vi "case structure.vi"() -> ()   [LabVIEW 2025]
panel:
  out "output":string
  in  "B":dbl
  in  "A":dbl
  out "Numeric":dbl
  in  "String 3":string
  out "month":string
  in  "month in num":dbl
  out "String":string
  in  "OK Button":bool
  in  "stop":bool
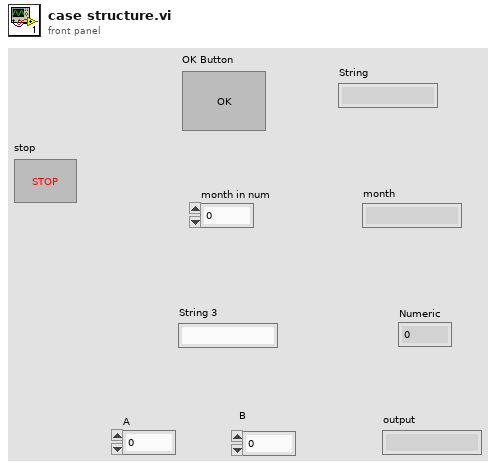
[diagram p1: front panel]
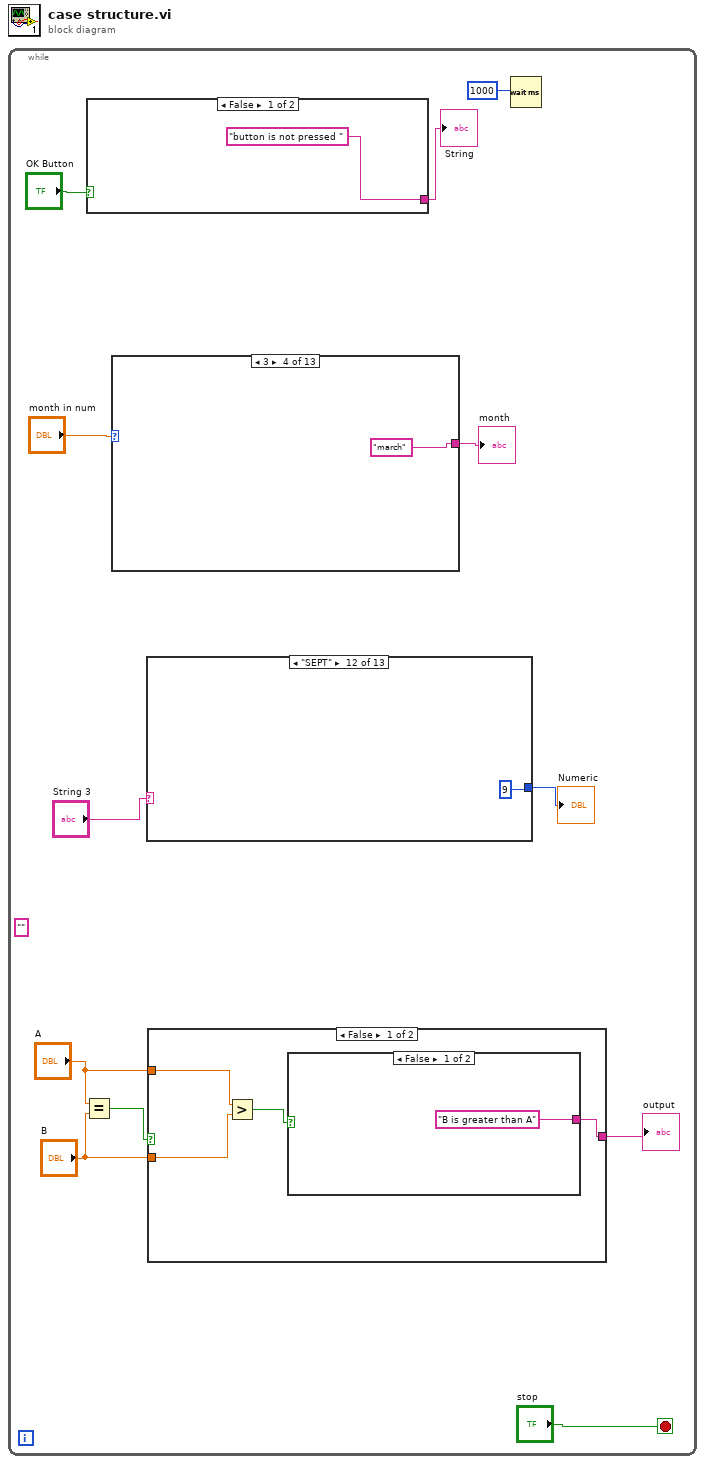
[diagram p0: block diagram]
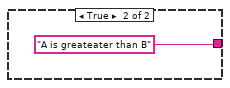
[diagram p2: hidden frame]
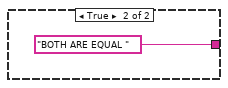
[diagram p3: hidden frame]
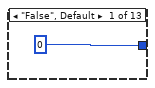
[diagram p4: hidden frame]
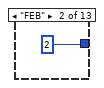
[diagram p5: hidden frame]
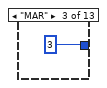
[diagram p6: hidden frame]
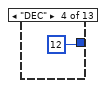
[diagram p7: hidden frame]
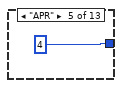
[diagram p8: hidden frame]
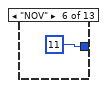
[diagram p9: hidden frame]
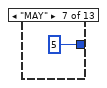
[diagram p10: hidden frame]
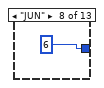
[diagram p11: hidden frame]
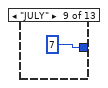
[diagram p12: hidden frame]
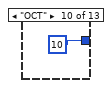
[diagram p13: hidden frame]
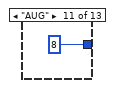
[diagram p14: hidden frame]
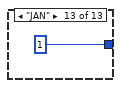
[diagram p15: hidden frame]
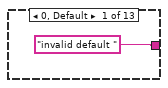
[diagram p16: hidden frame]
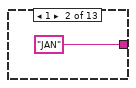
[diagram p17: hidden frame]
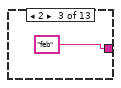
[diagram p18: hidden frame]
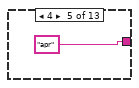
[diagram p19: hidden frame]
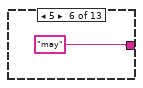
[diagram p20: hidden frame]
diagram:
  n1 = while {
    stop <- "stop" stop-if-true
    (unwired) "" ("String")
    n2 = Equal?(x="A", y="B") -> (x = y?=w4:bool)
    n3 = case shown="False" "OK Button" {
      tunnel: ["button is not pressed " "button is pressed "] -> w11
      frame False {
      }
      frame True {
      }
    }
    "String" <- w11
    n4 = case shown="3" "month in num" {
      tunnel: ["invalid default " "JAN" "feb" "march" "apr" "may" "jun" "july" "aug" "sept" "oct" "nov" "dec"] -> w7
      frame 0, Default {
      }
      frame 1 {
      }
      frame 2 {
      }
      frame 3 {
      }
      frame 4 {
      }
      frame 5 {
      }
      frame 6 {
      }
      frame 7 {
      }
      frame 8 {
      }
      frame 9 {
      }
      frame 10 {
      }
      frame 11 {
      }
      frame 12 {
      }
    }
    "month" <- w7
    n5 = case shown="\"SEPT\"" "String 3" {
      tunnel: [0 2 3 12 4 11 5 6 7 10 8 9 1] -> w5
      frame "False", Default {
      }
      frame "FEB" {
      }
      frame "MAR" {
      }
      frame "DEC" {
      }
      frame "APR" {
      }
      frame "NOV" {
      }
      frame "MAY" {
      }
      frame "JUN" {
      }
      frame "JULY" {
      }
      frame "OCT" {
      }
      frame "AUG" {
      }
      frame "SEPT" {
      }
      frame "JAN" {
      }
    }
    "Numeric" <- w5
    n6 = case shown="False" w4 {
      tunnel: [w13 "BOTH ARE EQUAL "] -> w1
      tunnel: "A" -> [w16 _]
      tunnel: "B" -> [w15 _]
      frame False {
        n7 = Greater?(x=w16, y=w15) -> (0:w14:bool)
        n8 = case shown="False" w14 {
          tunnel: ["B is greater than A" "A is greateater than B"] -> w13
          frame False {
          }
          frame True {
          }
        }
      }
      frame True {
      }
    }
    "output" <- w1
    n9 = Wait (ms)(milliseconds to wait=1000) -> ()  [unwired: 1 out]
  }
